vi "标定文件名选择.vi"() -> (3 "字符串":string)   [LabVIEW 2015]
panel:
  in  "选项卡控件":enum32{"选项卡 1"}(tab)
  in  "确定按钮":bool
  in  "组合框":string(combo)="G1机种"
  # "标定文件名选择界面"
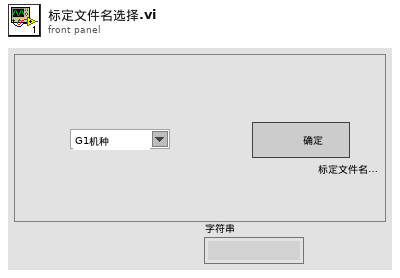
[diagram p1: front panel]
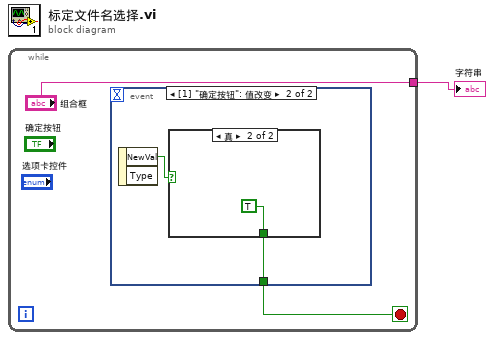
[diagram p0: block diagram]
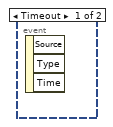
[diagram p2: hidden frame]
diagram:
  n1 = while {
    tunnel: ["组合框"] -> w1
    stop <- w3 stop-if-true
    n2 = event shown="[1] \"确定按钮\": 值改变" {
      selector: _ -> [_ _]
      dyn-events: _ -> [_ _]
      timeout: _ -> [_ _]
      tunnel: [_ w4] -> w3
      event Timeout {
        n3 = event-data() -> ()  [unwired: 1 in, 3 out]
      }
      event "确定按钮": Value Change {
        n4 = event-data() -> ("NewVal"=w5:bool)  [unwired: 1 in, 1 out]
        n5 = case shown="真" w5 {
          tunnel: [_ TRUE] -> w4
          frame False {
          }
          frame True {
          }
        }
      }
    }
  }
  "字符串" <- w1
